vi "WPI_GyroReset.vi"(8 "error in (no error)":errorcluster, 11 "GyroDevRef":T1) -> (0 "error out":errorcluster, 3 "GyroDevRef":T1)   [LabVIEW 2013]
doc: "Resets the gyroscope to a heading of zero. Use this VI to recalibrate the gyroscope after significant drift.\n\nThis software is licensed. Open the labview\\readme\\WPI Robotics Library Open Source License.txt file for more information."
uses:
  <vilib>/Rock Robotics/WPI/Gyro/WPI_GyroDevRef.ctl
  <vilib>/Rock Robotics/SystemInterfaces/Typedef/FPGA_TypedefAnalogModule.ctl
  <vilib>/Rock Robotics/SystemInterfaces/AI/FPGA_AIChannel.ctl
  <vilib>/Rock Robotics/SystemInterfaces/AI/FPGA_AIGyroChannel.ctl
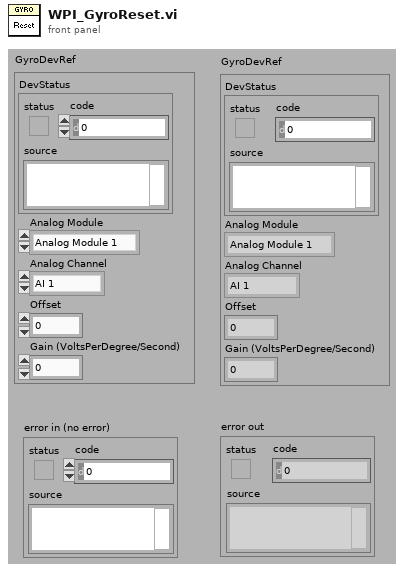
[diagram p1: front panel]
types:
  T1 = typedef "WPI_GyroDevRef.ctl" = cluster{"DevStatus":errorcluster, "Analog Module":T2, "Analog Channel":T3, "Offset":dbl, "Gain (VoltsPerDegree/Second)":dbl}
  T2 = typedef "FPGA_TypedefAnalogModule.ctl" = enum16{"Analog Module 1", "Analog Module 2"}
  T3 = typedef "FPGA_AIChannel.ctl" = enum8{"AI 1", "AI 2", "AI 3", "AI 4", "AI 5", "AI 6", "AI 7", "AI 8", "Invalid"}
  T4 = typedef "FPGA_AIGyroChannel.ctl" = enum8{"AI 1", "AI 2", "Invalid"}
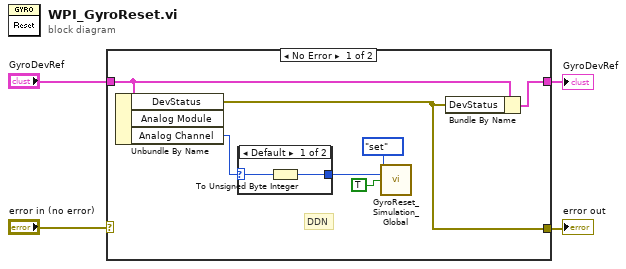
[diagram p0: block diagram]
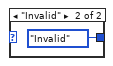
[diagram p2: hidden frame]
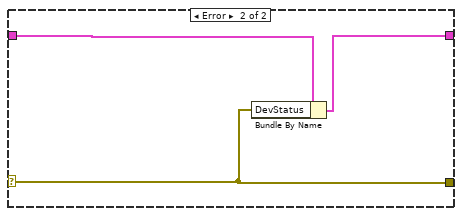
[diagram p3: hidden frame]
diagram:
  n1 = case shown="No Error" "error in (no error)" {
    selector: "error in (no error)" -> [_ w15]
    tunnel: "GyroDevRef" -> [w11 w17]
    tunnel: [w10 w16] -> w3
    tunnel: [w9 w15] -> w1
    frame No Error {
      # "DDN"
      n2 = Unbundle By Name(w11) -> ("DevStatus"=w9:errorcluster, "Analog Channel"=w8:T3)  [unwired: 1 out]
      n3 = case shown="Default" w8 {
        selector: w8 -> [w13 _]
        tunnel: [w12 FPGA_AIGyroChannel."Invalid" ("Analog Channel")] -> w5
        frame Default {
          n4 = To Unsigned Byte Integer(number=w13) -> (unsigned 8bit integer=w12:u8)
        }
        frame "Invalid" {
        }
      }
      n5 = call <vilib>:"GyroReset_Simulation_Global.vi"("menu"=enum16{"set", "get", "delete"}."set", "Gyro Channel"=w5, "reset in"=TRUE) -> ()  [unwired: 11 in, 2 out]
      n6 = Bundle By Name(cluster=w11, "DevStatus"=w9) -> (w10:T1)
    }
    frame Error {
      n7 = Bundle By Name(cluster=w17, "DevStatus"=w15) -> (w16:T1)
    }
  }
  "GyroDevRef" <- w3
  "error out" <- w1
